vi "FormatCloseReason.vi"(7 "error in (no error)":errorcluster, 8 "Send Reason (F)":bool, 9 "Reason":string, 10 "Status Code":T1 items=["Normal Closure"=1000, "Going Away"=1001, "Protocol Error"=1002, "Wrong Data Type"=1003, "Reserved 1004"=1004, "Reserved 1005"=1005, "Reserved 1006"=1006, "Non Consistent Data Type"=1007, "Policy Violation"=1008, "Message Too Big"=1009, "Extensions Negotiation Error"=1010, "Unexpected Condition"=1011, "Reserved 1015"=1015]) -> (0 "error out":errorcluster, 2 "Application Data":string)   [LabVIEW 2017, in "LV WebSockets.lvlib"]
uses:
  LV WebSockets.lvlib
  StatusCode.ctl
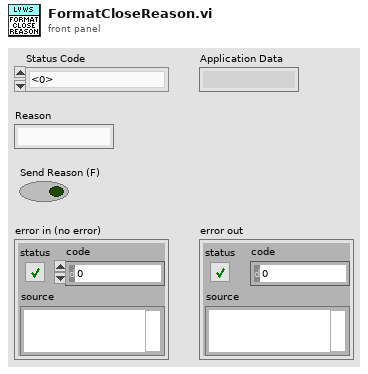
[diagram p1: front panel]
types:
  T1 = typedef "LV WebSockets.lvlib/StatusCode.ctl" = u16
  T2 = enum16{"big-endian, network order", "native, host order", "little-endian"}
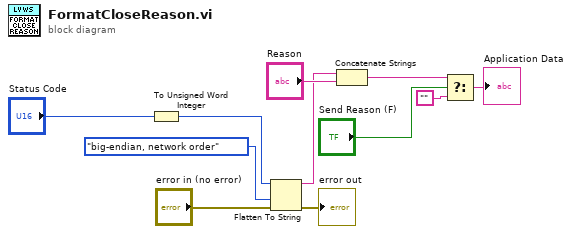
[diagram p0: block diagram]
diagram:
  n1 = To Unsigned Word Integer(number="Status Code") -> (unsigned 16bit integer=w2:T1)
  n2 = Flatten To String(anything=w2, byte order (0:big-endian, network order)=T2."big-endian, network order", error in (no error)="error in (no error)") -> (data string=w4:string, error out=→"error out":errorcluster)  [unwired: 1 in, 1 out]
  n3 = Concatenate Strings(w4, "Reason") -> (w6:string)
  n4 = Select(t=w6, s="Send Reason (F)", f="") -> (s? t:f=→"Application Data":string)
